vi "Teleop.vi"(10 "Match Info":T1={"Autonomous Elapsed Seconds"=0.0, "TeleOp Elapsed Seconds"=0.0, "Disabled Elapsed Seconds"=0.0, "Visited Autonomous"=FALSE, "Visited TeleOp"=FALSE, "Visited Disabled"=FALSE, "Autonomous Settings"={"Autonomous Style"=enum."Independent", "VI Refnum"=refnum}}, 11 "Call Context":T2) -> ()   [LabVIEW 2020]
doc: "This VI is called for each TeleOp packet received from the DS where the robot is not disabled. It is often used to read from the joysticks and update I/O or to update setpoints for timed control loops. It should complete and return within 20 milliseconds or it may miss DS packets."
uses:
  <vilib>/Rock Robotics/WPI/DriverStation/WPI_DriverStationDerivedRobotMode.ctl
  <vilib>/Rock Robotics/WPI/DriverStation/WPI_DriverStationMatch Info.ctl
  <vilib>/Rock Robotics/WPI/ThirdParty/Phoenix-LabVIEW/Motor Controller/Controls/CTRE_Phoenix_MotorControl_ControlMode.ctl
  <vilib>/Rock Robotics/WPI/ThirdParty/REV Robotics/REVLib/Typedef/Spark MAX Control Type.ctl
  <vilib>/Rock Robotics/Network Tables/NT Read Boolean.vi
  <vilib>/Rock Robotics/Network Tables/NT Read Number.vi
  <vilib>/Rock Robotics/WPI/Utilities/WPI_GetSetVariantRefNum.vi
  <vilib>/Rock Robotics/Network Tables/NT Write Boolean Array.vi
  <vilib>/Rock Robotics/Network Tables/NT Write Numeric Array.vi
  981LabViewComponents/2022 Robot Global Data.vi
panel:
  out "command to\nset output":dbl
  in  "multiper for arm speed":dbl=0.1
  out "Sensor Position":dbl
  out "element":dbl
  out "x-y":dbl
  out "coerced(x)":dbl
  out "Joystick1":dbl(slide) scale=-1.0..1.0
  out "Joystick0":dbl(slide) scale=-1.0..1.0
  out "Sample Slider 0":dbl(slide) scale=0.0..5.0
  out "Sample Boolean 1":bool
  out "Sample Boolean 0":bool
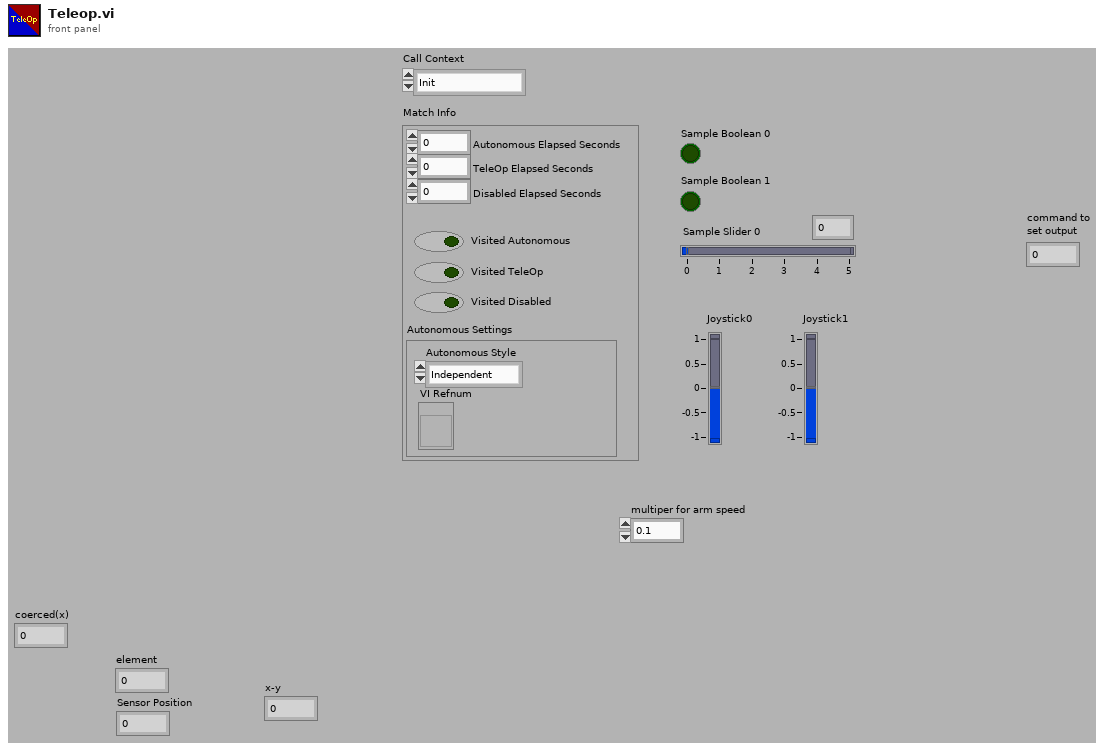
[diagram p1: front panel]
types:
  T1 = typedef "WPI_DriverStationMatch Info.ctl" = cluster{"Autonomous Elapsed Seconds":dbl, "TeleOp Elapsed Seconds":dbl, "Disabled Elapsed Seconds":dbl, "Visited Autonomous":bool, "Visited TeleOp":bool, "Visited Disabled":bool, "Autonomous Settings":cluster{"Autonomous Style":enum16{"Iterative", "Independent"}, "VI Refnum":refnum<vi>}}
  T2 = typedef "WPI_DriverStationDerivedRobotMode.ctl" = enum16{"Init", "Execute", "Stop"}
  T3 = typedef "Spark MAX Control Type.ctl" = enum16{"Percent VBus", "Voltage", "Velocity", "Position", "Smart Motion", "Current", "Smart Velocity"}
  T4 = typedef "CTRE_Phoenix_MotorControl_ControlMode.ctl" = u16
  T5 = typedef "WPI_JoystickDevRef.ctl" = cluster{"Device":T6}
  T6 = typedef "WPI_JoystickDeviceEnum.ctl" = enum16{"USB 0", "USB 1", "USB 2", "USB 3", "USB 4", "USB 5"}
  T7 = typedef "WPI_RobotDriveDevRef.ctl" = cluster{"DevStatus":errorcluster, "Motors[]":T8[], "Square Inputs":bool, "Max Output":dbl}
  T8 = typedef "WPI_MotorControlDeviceRef.ctl" = cluster{"DeviceStatus":errorcluster, "Type":T9, "PWM":cluster{"PWM Channel":T10, "DeadBand":T11}, "CAN":cluster{"Device Number":u8, "SetOutput VI Ref":variant, "GetOutput VI Ref":variant, "Enable VI Ref":variant, "Disable VI Ref":variant, "Data":variant}, "Invert":bool, "DIO PWM":cluster{"PWM \"Enable\" Channel":T10, "DIOChannel":T12, "PWM Rate":dbl}}
  T9 = typedef "WPI_MotorControlType.ctl" = enum16{"PWM", "CAN", "DIO PWM"}
  T10 = typedef "FPGA_DIOPWMChannel.ctl" = enum8{"PWM 0", "PWM 1", "PWM 2", "PWM 3", "PWM 4", "PWM 5", "PWM 6", "PWM 7", "PWM 8", "PWM 9", "PWM MXP 0", "PWM MXP 1", "PWM MXP 2", "PWM MXP 3", "PWM MXP 4", "PWM MXP 5", "PWM MXP 6", "PWM MXP 7", "PWM MXP 8", "PWM MXP 9", "Invalid"}
  T11 = typedef "WPI_PWMDeadband.ctl" = cluster{"Name":string, "maxPositivePwm":i32, "minPositivePwm":i32, "centerPwm":i32, "maxNegativePwm":i32, "minNegativePwm":i32, "angularRange":u16}
  T12 = typedef "FPGA_DIOChannel.ctl" = enum8{"DIO 0", "DIO 1", "DIO 2", "DIO 3", "DIO 4", "DIO 5", "DIO 6", "DIO 7", "DIO 8", "DIO 9", "DIO MXP 0", "DIO MXP 1", "DIO MXP 2", "DIO MXP 3", "DIO MXP 4", "DIO MXP 5", "DIO MXP 6", "DIO MXP 7", "DIO MXP 8", "DIO MXP 9", "DIO MXP 10", "DIO MXP 11", "DIO MXP 12", "DIO MXP 13", "DIO MXP 14", "DIO MXP 15", "SPI Port CS1", "SPI Port CS2", "SPI Port CS3", "SPI Port MISO", "SPI Port MOSI", "Invalid"}
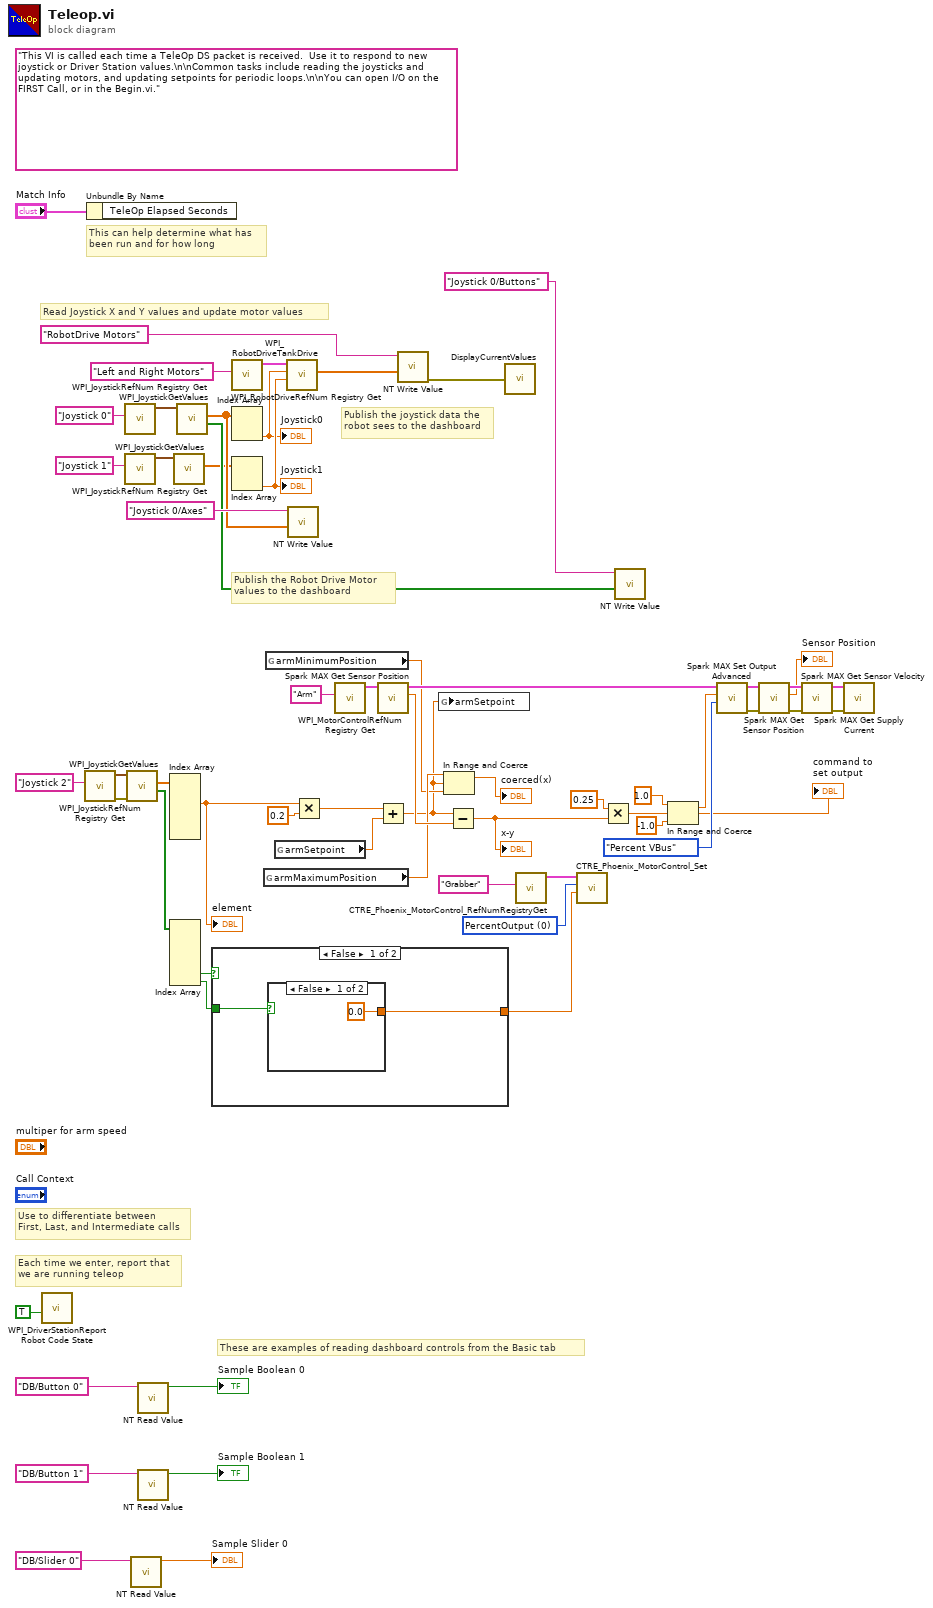
[diagram p0: block diagram]
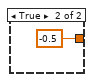
[diagram p2: hidden frame]
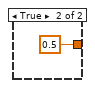
[diagram p3: hidden frame]
diagram:
  w38 = T4 0 items=["PercentOutput"=0, "Position"=1, "Velocity"=2, "Current"=3, "Follower"=5, "MotionProfile"=6, "MotionMagic"=7, "MotionProfileArc"=10, "Disabled"=15] ("Control Mode")
  (unwired) "This VI is called each time a TeleOp DS packet is received.  Use it to respond to new joystick or Driver Station values.\n\nCommon tasks include reading the joysticks and updating motors, and updating setpoints for periodic loops.\n\nYou can open I/O on the FIRST Call, or in the Begin.vi."
  # "Publish the Robot Drive Motor\nvalues to the dashboard"
  # "Publish the joystick data the\nrobot sees to the dashboard"
  # "These are examples of reading dashboard controls from the Basic tab"
  # "Each time we enter, report that\nwe are running teleop"
  # "Use to differentiate between\nFirst, Last, and Intermediate calls"
  # "This can help determine what has\nbeen run and for how long"
  # "Read Joystick X and Y values and update motor values"
  n1 = call <vilib>:"WPI_DriverStationReport Robot Code State.vi"("TeleOp"=TRUE ("Autonomous")) -> ()  [unwired: 10 in, 1 out]
  n2 = call <vilib>:"WPI_JoystickRefNum Registry Get.vi"("refnum name"="Joystick 2") -> ("error out"=w32:errorcluster, "JoystickDevRef"=w33:T5)  [unwired: 1 in, 8 out]
  n3 = Unbundle By Name("Match Info") -> ()  [unwired: 1 out]
  n4 = call <vilib>:"WPI_JoystickRefNum Registry Get.vi"("refnum name"="Joystick 0") -> ("JoystickDevRef"=w50:T5)  [unwired: 1 in, 9 out]
  n5 = call <vilib>:"WPI_JoystickRefNum Registry Get.vi"("refnum name"="Joystick 1") -> ("JoystickDevRef"=w42:T5)  [unwired: 1 in, 9 out]
  n6 = call <vilib>:"WPI_JoystickGetValues.vi"("error in (no error)"=w32, "JoystickDevRef"=w33) -> ("Buttons"=w31:bool[], "Axes"=w28:dbl[])  [unwired: 5 in, 3 out]
  n7 = call-poly <vilib>:"NT Read Value.vi"("Name"="DB/Slider 0" ("refnum name")) -> ("Numeric"=→"Sample Slider 0":dbl)  [unwired: 9 in, 1 out]
  n8 = call-poly <vilib>:"NT Read Value.vi"("Name"="DB/Button 0" ("refnum name")) -> ("Boolean"=→"Sample Boolean 0":bool)  [unwired: 9 in, 1 out]
  n9 = call-poly <vilib>:"NT Read Value.vi"("Name"="DB/Button 1" ("refnum name")) -> ("Boolean"=→"Sample Boolean 1":bool)  [unwired: 9 in, 1 out]
  n10 = Index Array(array=w28) -> (element #2=w5:dbl)  [unwired: 6 in, 5 out]
  "element" <- w5
  n11 = Index Array(array=w31) -> (element #5=w30:bool, element #6=w29:bool)  [unwired: 6 in, 4 out]
  n12 = call <vilib>:"WPI_JoystickGetValues.vi"("JoystickDevRef"=w42) -> ("Axes"=w41:dbl[])  [unwired: 6 in, 4 out]
  n13 = call <vilib>:"WPI_JoystickGetValues.vi"("JoystickDevRef"=w50) -> ("Buttons"=w46:bool[], "Axes"=w47:dbl[])  [unwired: 6 in, 3 out]
  n14 = case shown="False" w30 {
    tunnel: [w62 0.5] -> w27
    tunnel: w29 -> [w63 _]
    frame False {
      n15 = case shown="False" w63 {
        tunnel: [0.0 -0.5] -> w62
        frame False {
        }
        frame True {
        }
      }
    }
    frame True {
    }
  }
  n16 = call <vilib>:"WPI_RobotDriveRefNum Registry Get.vi"("refnum name"="Left and Right Motors") -> ("RobotDriveDevRef"=w52:T7)  [unwired: 1 in, 9 out]
  n17 = Index Array(array=w47) -> (element #2=w35:dbl)  [unwired: 2 in, 1 out]
  "Joystick0" <- w35
  n18 = Index Array(array=w41) -> (element #2=w36:dbl)  [unwired: 2 in, 1 out]
  "Joystick1" <- w36
  n19 = global read "2022 Robot Global Data.vi" "armMaximumPosition"() -> (w11:dbl)
  n20 = global read "2022 Robot Global Data.vi" "armMinimumPosition"() -> (w10:dbl)
  n21 = global read "2022 Robot Global Data.vi" "armSetpoint"() -> (w7:dbl)
  n22 = call <vilib>:"WPI_RobotDriveTankDrive.vi"("Right axis value"=w36, "Left axis value"=w35, "RobotDriveDevRef"=w52) -> ("Motor Values"=w45:dbl[])  [unwired: 6 in, 2 out]
  n23 = call-poly <vilib>:"NT Write Value.vi"("Numeric Array"=w47, "Name"="Joystick 0/Axes") -> ()  [unwired: 9 in, 1 out]
  n24 = Multiply(x=w5, y=0.2) -> (x*y=w8:dbl)
  n25 = call <vilib>:"WPI_MotorControlRefNum Registry Get.vi"("refnum name"="Arm") -> ("MotorControlDevRef"=w3:T8)  [unwired: 9 in, 1 out]
  n26 = call <vilib>:"Spark MAX Get Sensor Position.vi"("MotorControlDevRef in"=w3) -> ("Sensor Position"=w20:dbl, "MotorControlDevRef out"=w15:T8)  [unwired: 7 in, 2 out]
  n27 = Add(x=w8, y=w7) -> (x+y=w2:dbl)
  n28 = call-poly <vilib>:"NT Write Value.vi"("Numeric Array"=w45, "Name"="RobotDrive Motors") -> ("error out"=w40:errorcluster)  [unwired: 9 in]
  n29 = global write "2022 Robot Global Data.vi" "armSetpoint"(w2) -> ()
  n30 = In Range and Coerce(upper limit=w11, x=w2, lower limit=w10) -> (coerced(x)=→"coerced(x)":dbl)  [unwired: 1 out]
  n31 = Subtract(x=w2, y=w20) -> (x-y=w19:dbl)
  "x-y" <- w19
  n32 = call "DisplayCurrentValues.vi"("error in (no error)"=w40) -> ()  [unwired: 5 out]
  n33 = call <vilib>:"CTRE_Phoenix_MotorControl_RefNumRegistryGet.vi"("refnum name"="Grabber") -> ("PhoenixMotorControlDevRef"=w39:T8)  [unwired: 9 in, 1 out]
  n34 = call <vilib>:"CTRE_Phoenix_MotorControl_Set.vi"("Output"=w27, "Control Mode"=w38, "PhoenixMotorControlDevRef"=w39) -> ()  [unwired: 7 in, 2 out]
  n35 = Multiply(x=0.25, y=w19) -> (x*y=w16:dbl)
  "command to\nset output" <- w16
  n36 = call-poly <vilib>:"NT Write Value.vi"("Boolean Array"=w46, "Name"="Joystick 0/Buttons") -> ()  [unwired: 9 in, 1 out]
  n37 = In Range and Coerce(upper limit=1.0, x=w16, lower limit=-1.0) -> (coerced(x)=w12:dbl)  [unwired: 1 out]
  n38 = call <vilib>:"Spark MAX Set Output Advanced.vi"("Control Mode"=Spark_MAX_Control_Type."Percent VBus", "Setpoint"=w12, "MotorControlDevRef"=w15) -> ("error out"=w13:errorcluster, "MotorControlDevRef"=w14:T8)  [unwired: 7 in]
  n39 = call <vilib>:"Spark MAX Get Sensor Position.vi"("error in (no error)"=w13, "MotorControlDevRef in"=w14) -> ("error out"=w25:errorcluster, "Sensor Position"=→"Sensor Position":dbl, "MotorControlDevRef out"=w24:T8)  [unwired: 6 in, 1 out]
  n40 = call <vilib>:"Spark MAX Get Sensor Velocity.vi"("error in (no error)"=w25, "MotorControlDevRef in"=w24) -> ("error out"=w21:errorcluster, "MotorControlDevRef out"=w22:T8)  [unwired: 6 in, 2 out]
  n41 = call <vilib>:"Spark MAX Get Supply Current.vi"("error in (no error)"=w21, "MotorControlDevRef in"=w22) -> ()  [unwired: 6 in, 4 out]
